vi "Graphics-Draw Box.vi"(3 "H":dbl=1.0, 4 "Y":dbl, 5 "Width":dbl=1.0, 6 "X":dbl) -> (1 "output cluster":cluster{dbl[], dbl[]})   [LabVIEW 2015]
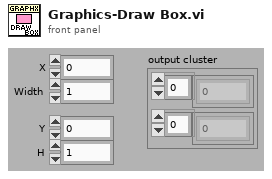
[diagram p1: front panel]
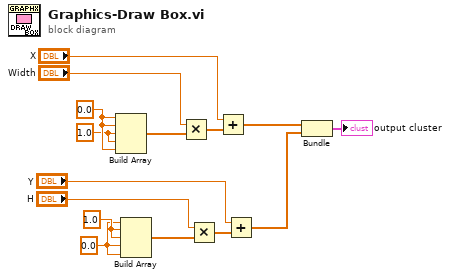
[diagram p0: block diagram]
diagram:
  w12 = 1.0
  w13 = 0.0
  w15 = 1.0
  w14 = 0.0
  n1 = Build Array(w13, w13, w12, w12, w13) -> (w11:dbl[])
  n2 = Build Array(w14, w15, w15, w14, w14) -> (w6:dbl[])
  n3 = Multiply(x="Width", y=w11) -> (x*y=w9:dbl[])
  n4 = Multiply(x="H", y=w6) -> (x*y=w7:dbl[])
  n5 = Add(x="X", y=w9) -> (x+y=w3:dbl[])
  n6 = Add(x="Y", y=w7) -> (x+y=w2:dbl[])
  n7 = Bundle(w3, w2) -> (→"output cluster":cluster{dbl[], dbl[]})  [unwired: 1 in]
